vi "File Info Test.vi"() -> ()   [LabVIEW 2021, in "Test Files.lvlib"]
uses:
  Test Files.lvlib
  CustomSortPath.lvlib
  <vilib>/addons/_JKI Toolkits/Caraya/classes/Test/Test.lvclass
  <vilib>/addons/_JKI Toolkits/Caraya/classes/Assert/Assert.lvclass
  <vilib>/addons/_JKI Toolkits/Caraya/classes/Assert/Assert Equal Value_Variant.vi
panel:
  out "error out":errorcluster
  in  "error in (no error)":errorcluster
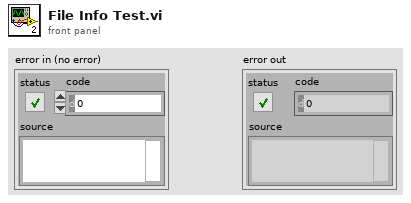
[diagram p1: front panel]
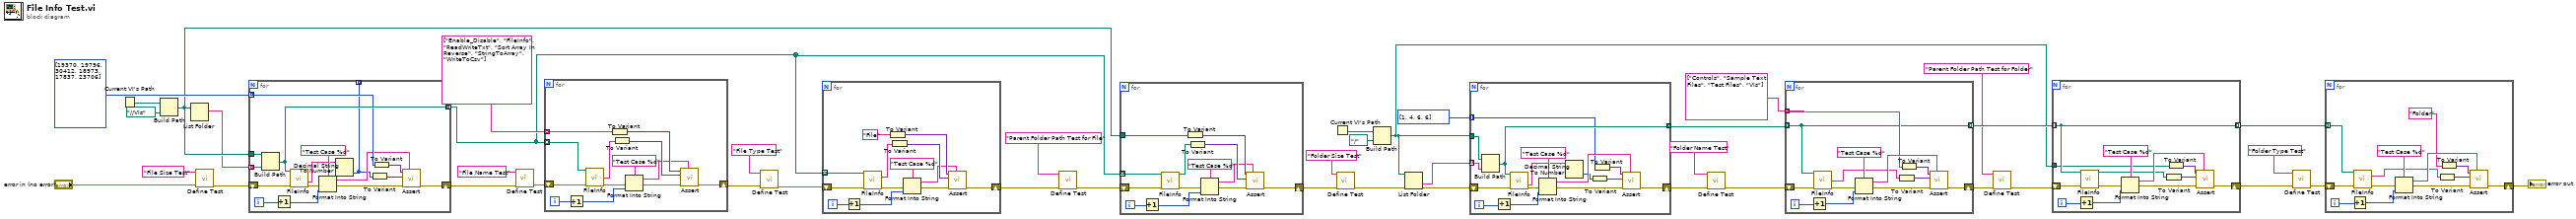
[diagram p0: block diagram]
diagram:
  n1 = Current VI's Path() -> (path=w42:path)
  n2 = Build Path(base path=w42, name or relative path=path "../../VIs") -> (appended path=w26:path)
  n3 = List Folder(path=w26) -> (filenames=w1:string[])  [unwired: 3 in, 3 out]
  n4 = call <vilib>:"Define Test.vi"("error in (no error)"="error in (no error)", "Label (VI Title)"="File Size Test") -> ("error out"=w39:errorcluster)  [unwired: 8 in, 1 out]
  n5 = for {
    tunnel: w26 -> [w58]
    tunnel: w1 -> [w57] mode=indexing
    tunnel: [w54] -> w27 mode=indexing
    tunnel: i64[] [19370, 19796, 30412, 18973, 17837, 23706] -> [w53] mode=indexing
    shift-right: [w52] -> w37
    shift-left: w39 -> [w56]
    tunnel: [w45] -> _ mode=indexing
    i -> [w50]
    n6 = Build Path(base path=w58, name or relative path=w57) -> (appended path=w54:path)
    n7 = Increment(x=w50) -> (x+1=w49:i32)
    n8 = call "FileInfo.vi"("File/Folder Path"=w54, "error in (no error)"=w56) -> ("Size"=w47:string, "error out"=w55:errorcluster)  [unwired: 9 in, 3 out]
    n9 = Format Into String(format string="Test Case %d", error in=w55, w49) -> (resulting string=w46:string, error out=w51:errorcluster)  [unwired: 1 in]
    n10 = Decimal String To Number(string=w47) -> (number=w45:i32)  [unwired: 2 in, 1 out]
    n11 = To Variant(anything=w45) -> (Variant=w43:variant)
    n12 = To Variant(anything=w53) -> (Variant=w44:variant)
    n13 = call-poly <vilib>:"Assert.vi"("Label"=w46, "error in (no error)"=w51, "Y"=w43, "X"=w44) -> ("error out"=w52:errorcluster)  [unwired: 6 in, 1 out]
  }
  n14 = call <vilib>:"Define Test.vi"("error in (no error)"=w37, "Label (VI Title)"="File Name Test") -> ("error out"=w36:errorcluster)  [unwired: 8 in, 1 out]
  n15 = for {
    shift-right: [w67] -> w33
    shift-left: w36 -> [w71]
    tunnel: w27 -> [w66] mode=indexing
    tunnel: string[] ["Enable_Disable", "FileInfo", "ReadWriteTxt", "Sort Array In Reverse", "StringToArray", "WriteToCsv"] -> [w64] mode=indexing
    i -> [w63]
    n16 = Increment(x=w63) -> (x+1=w60:i32)
    n17 = call "FileInfo.vi"("File/Folder Path"=w66, "error in (no error)"=w71) -> ("Name"=w65:string, "error out"=w70:errorcluster)  [unwired: 9 in, 3 out]
    n18 = To Variant(anything=w64) -> (Variant=w68:variant)
    n19 = To Variant(anything=w65) -> (Variant=w69:variant)
    n20 = Format Into String(format string="Test Case %d", error in=w70, w60) -> (resulting string=w59:string, error out=w62:errorcluster)  [unwired: 1 in]
    n21 = call-poly <vilib>:"Assert.vi"("Label"=w59, "error in (no error)"=w62, "Y"=w69, "X"=w68) -> ("error out"=w67:errorcluster)  [unwired: 6 in, 1 out]
  }
  n22 = call <vilib>:"Define Test.vi"("error in (no error)"=w33, "Label (VI Title)"="File Type Test") -> ("error out"=w32:errorcluster)  [unwired: 8 in, 1 out]
  n23 = for {
    shift-right: [w80] -> w30
    shift-left: w32 -> [w84]
    tunnel: w27 -> [w73] mode=indexing
    i -> [w79]
    n24 = Increment(x=w79) -> (x+1=w76:i32)
    n25 = call "FileInfo.vi"("File/Folder Path"=w73, "error in (no error)"=w84) -> ("Type"=w75:string, "error out"=w83:errorcluster)  [unwired: 9 in, 3 out]
    n26 = To Variant(anything="File" ("Type")) -> (Variant=w81:variant)
    n27 = To Variant(anything=w75) -> (Variant=w82:variant)
    n28 = Format Into String(format string="Test Case %d", error in=w83, w76) -> (resulting string=w72:string, error out=w78:errorcluster)  [unwired: 1 in]
    n29 = call-poly <vilib>:"Assert.vi"("Label"=w72, "error in (no error)"=w78, "Y"=w82, "X"=w81) -> ("error out"=w80:errorcluster)  [unwired: 6 in, 1 out]
  }
  n30 = call <vilib>:"Define Test.vi"("error in (no error)"=w30, "Label (VI Title)"="Parent Folder Path Test for File") -> ("error out"=w28:errorcluster)  [unwired: 8 in, 1 out]
  n31 = for {
    shift-right: [w93] -> w17
    shift-left: w28 -> [w97]
    tunnel: w27 -> [w88] mode=indexing
    tunnel: w26 -> [w87]
    i -> [w92]
    n32 = Increment(x=w92) -> (x+1=w89:i32)
    n33 = call "FileInfo.vi"("File/Folder Path"=w88, "error in (no error)"=w97) -> ("ParentFolderPath"=w86:path, "error out"=w96:errorcluster)  [unwired: 9 in, 3 out]
    n34 = To Variant(anything=w87) -> (Variant=w94:variant)
    n35 = To Variant(anything=w86) -> (Variant=w95:variant)
    n36 = Format Into String(format string="Test Case %d", error in=w96, w89) -> (resulting string=w85:string, error out=w91:errorcluster)  [unwired: 1 in]
    n37 = call-poly <vilib>:"Assert.vi"("Label"=w85, "error in (no error)"=w91, "Y"=w95, "X"=w94) -> ("error out"=w93:errorcluster)  [unwired: 6 in, 1 out]
  }
  n38 = Current VI's Path() -> (path=w23:path)
  n39 = call <vilib>:"Define Test.vi"("error in (no error)"=w17, "Label (VI Title)"="Folder Size Test") -> ("error out"=w19:errorcluster)  [unwired: 8 in, 1 out]
  n40 = Build Path(base path=w23, name or relative path=path "../..") -> (appended path=w2:path)
  n41 = List Folder(path=w2, error in=w19) -> (folder names=w21:string[], error out=w22:errorcluster)  [unwired: 2 in, 2 out]
  n42 = for {
    tunnel: [w111] -> w15 mode=indexing
    shift-right: [w110] -> w14
    shift-left: w22 -> [w113]
    tunnel: w21 -> [w102] mode=indexing
    tunnel: w2 -> [w103]
    tunnel: i64[] [1, 4, 6, 6] ("number") -> [w101] mode=indexing
    i -> [w108]
    n43 = Build Path(base path=w103, name or relative path=w102) -> (appended path=w111:path)
    n44 = Increment(x=w108) -> (x+1=w107:i32)
    n45 = call "FileInfo.vi"("File/Folder Path"=w111, "error in (no error)"=w113) -> ("Size"=w105:string, "error out"=w112:errorcluster)  [unwired: 9 in, 3 out]
    n46 = Format Into String(format string="Test Case %d", error in=w112, w107) -> (resulting string=w104:string, error out=w109:errorcluster)  [unwired: 1 in]
    n47 = Decimal String To Number(string=w105) -> (number=w100:i32)  [unwired: 2 in, 1 out]
    n48 = To Variant(anything=w100) -> (Variant=w99:variant)
    n49 = To Variant(anything=w101) -> (Variant=w98:variant)
    n50 = call-poly <vilib>:"Assert.vi"("Label"=w104, "error in (no error)"=w109, "Y"=w99, "X"=w98) -> ("error out"=w110:errorcluster)  [unwired: 6 in, 1 out]
  }
  n51 = call <vilib>:"Define Test.vi"("error in (no error)"=w14, "Label (VI Title)"="Folder Name Test") -> ("error out"=w13:errorcluster)  [unwired: 8 in, 1 out]
  n52 = for {
    shift-right: [w122] -> w10
    shift-left: w13 -> [w126]
    tunnel: string[] ["Controls", "Sample Text Files", "Test Files", "VIs"] -> [w116] mode=indexing
    tunnel: w15 -> [w114] mode=indexing
    tunnel: [w114] -> w11 mode=indexing
    i -> [w120]
    n53 = Increment(x=w120) -> (x+1=w119:i32)
    n54 = call "FileInfo.vi"("File/Folder Path"=w114, "error in (no error)"=w126) -> ("Name"=w115:string, "error out"=w125:errorcluster)  [unwired: 9 in, 3 out]
    n55 = Format Into String(format string="Test Case %d", error in=w125, w119) -> (resulting string=w117:string, error out=w121:errorcluster)  [unwired: 1 in]
    n56 = To Variant(anything=w115) -> (Variant=w124:variant)
    n57 = To Variant(anything=w116) -> (Variant=w123:variant)
    n58 = call-poly <vilib>:"Assert.vi"("Label"=w117, "error in (no error)"=w121, "Y"=w124, "X"=w123) -> ("error out"=w122:errorcluster)  [unwired: 6 in, 1 out]
  }
  n59 = call <vilib>:"Define Test.vi"("error in (no error)"=w10, "Label (VI Title)"="Parent Folder Path Test for Folder") -> ("error out"=w9:errorcluster)  [unwired: 8 in, 1 out]
  n60 = for {
    shift-right: [w135] -> w6
    shift-left: w9 -> [w139]
    tunnel: w11 -> [w129] mode=indexing
    tunnel: [w129] -> w7 mode=indexing
    tunnel: w2 -> [w127]
    i -> [w133]
    n61 = Increment(x=w133) -> (x+1=w132:i32)
    n62 = call "FileInfo.vi"("File/Folder Path"=w129, "error in (no error)"=w139) -> ("ParentFolderPath"=w128:path, "error out"=w138:errorcluster)  [unwired: 9 in, 3 out]
    n63 = Format Into String(format string="Test Case %d", error in=w138, w132) -> (resulting string=w130:string, error out=w134:errorcluster)  [unwired: 1 in]
    n64 = To Variant(anything=w128) -> (Variant=w137:variant)
    n65 = To Variant(anything=w127) -> (Variant=w136:variant)
    n66 = call-poly <vilib>:"Assert.vi"("Label"=w130, "error in (no error)"=w134, "Y"=w137, "X"=w136) -> ("error out"=w135:errorcluster)  [unwired: 6 in, 1 out]
  }
  n67 = call <vilib>:"Define Test.vi"("error in (no error)"=w6, "Label (VI Title)"="Folder Type Test") -> ("error out"=w5:errorcluster)  [unwired: 8 in, 1 out]
  n68 = for {
    shift-right: [w148] -> w3
    shift-left: w5 -> [w152]
    tunnel: w7 -> [w142] mode=indexing
    i -> [w146]
    n69 = Increment(x=w146) -> (x+1=w145:i32)
    n70 = call "FileInfo.vi"("File/Folder Path"=w142, "error in (no error)"=w152) -> ("Type"=w140:string, "error out"=w151:errorcluster)  [unwired: 9 in, 3 out]
    n71 = Format Into String(format string="Test Case %d", error in=w151, w145) -> (resulting string=w143:string, error out=w147:errorcluster)  [unwired: 1 in]
    n72 = To Variant(anything=w140) -> (Variant=w150:variant)
    n73 = To Variant(anything="Folder" ("format string")) -> (Variant=w149:variant)
    n74 = call-poly <vilib>:"Assert.vi"("Label"=w143, "error in (no error)"=w147, "Y"=w150, "X"=w149) -> ("error out"=w148:errorcluster)  [unwired: 6 in, 1 out]
  }
  "error out" <- w3
